vi "Write Password.vi"(8 "Error In":errorcluster, 10 "Password":string, 11 "BNT_BlowfishFactory in":refnum<class "BNT_BlowfishFactory.lvclass">) -> (0 "Error Out":errorcluster, 3 "BNT_BlowfishFactory out":refnum<class "BNT_BlowfishFactory.lvclass">)   [LabVIEW 2018, in "BNT_Factories.lvlib" / "BNT_BlowfishFactory.lvclass"]
uses:
  BNT_BlowfishFactory.lvclass
  BNT_BlowfishFactory.lvclass/BNT_BlowfishFactory.ctl
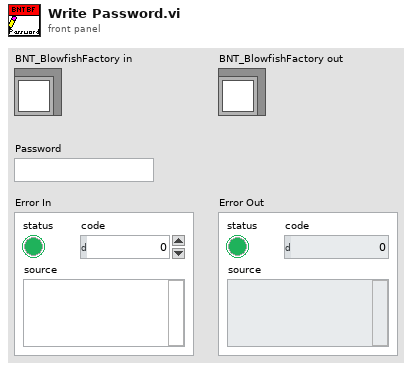
[diagram p1: front panel]
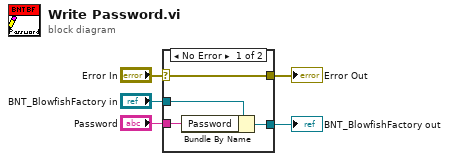
[diagram p0: block diagram]
diagram:
  n1 = case shown="No Error" "Error In" {
    selector: "Error In" -> [w9 w10]
    tunnel: [w9 w10] -> w2
    tunnel: [w7 w11] -> w4
    tunnel: "BNT_BlowfishFactory in" -> [w8 w11]
    tunnel: "Password" -> [w6 _]
    frame No Error {
      n2 = Bundle By Name(cluster=w8, "Password"=w6) -> (w7:refnum<class "BNT_BlowfishFactory.lvclass">)
    }
    frame Error {
    }
  }
  "BNT_BlowfishFactory out" <- w4
  "Error Out" <- w2
